vi "Greyscale Image to ARGB Image.vi"(8 "error in (no error)":errorcluster, 10 "ARGB Image Destination in":T1, 11 "Greyscale Image Source in":T2) -> (0 "error out":errorcluster, 3 "ARGB Image Destination":T1)   [LabVIEW 2020, in "image.lvlib"]
doc: "Convert a Greyscale Image to an ARGB Image. The ARGB Image Destination will be sized to fit the Greyscale Source Image."
uses:
  image.lvlib
  ARGB Image.ctl
  Greyscale Image.ctl
  common/common.lvlib
  common/bin/gartoolkit_32-1.dll
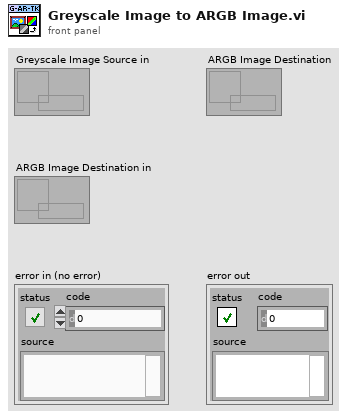
[diagram p1: front panel]
types:
  T1 = typedef "image.lvlib/ARGB Image.ctl" = refnum<data-value>
  T2 = typedef "image.lvlib/Greyscale Image.ctl" = refnum<data-value>
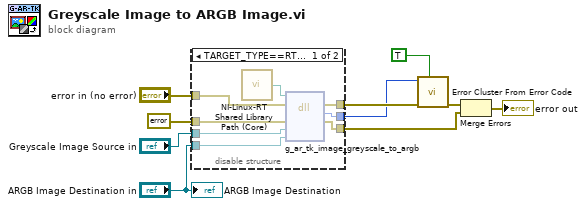
[diagram p0: block diagram]
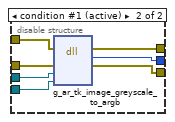
[diagram p2: hidden frame]
diagram:
  n1 = disable-structure shown="TARGET_TYPE==RT&&OS==Linux" {
    disable-tunnel: "error in (no error)" -> [w17 w25]
    disable-tunnel: errorcluster {"status"=FALSE, "code"=0, "source"=""} ("error constant") -> [w16 w24]
    disable-tunnel: "Greyscale Image Source in" -> [w15 w23]
    disable-tunnel: "ARGB Image Destination in" -> [w14 w22]
    disable-tunnel: [w13 w21] -> w4
    disable-tunnel: [w12 w20] -> w3
    disable-tunnel: [w11 w19] -> w2
    frame condition #0 {
      n2 = call "NI-Linux-RT Shared Library Path (Core).vi"() -> ("Path"=w18:path)
      n3 = dll-call lib="?" fn="g_ar_tk_image_greyscale_to_argb"(path in=w18, error in=w17, "error_cluster"=w16, "EDVR src"=w15, "EDVR dst"=w14) -> (error out=w13:errorcluster, w12:i32, "error_cluster"=w11:errorcluster)  [unwired: 3 in, 1 out]
    }
    frame condition #1 (active) {
      n4 = dll-call lib="C:/serenial/lib/g-augmented-reality-toolkit/LabVIEW/common/bin/gartoolkit_*-1.*" fn="g_ar_tk_image_greyscale_to_argb"(error in=w25, "error_cluster"=w24, "EDVR src"=w23, "EDVR dst"=w22) -> (error out=w21:errorcluster, w20:i32, "error_cluster"=w19:errorcluster)  [unwired: 4 in, 1 out]
    }
  }
  n5 = call <vilib>:"Error Cluster From Error Code.vi"("show call chain? (False)"=TRUE, "error in (no error)"=w4, "error code (0)"=w3) -> ("error out"=w9:errorcluster)  [unwired: 6 in]
  n6 = Merge Errors(w9, w2) -> (→"error out":errorcluster)
  "ARGB Image Destination" <- "ARGB Image Destination in"
